vi "ToPythonVersionString.vi"(11 "Python版本":T1) -> (3 "python版本字符串":string)   [LabVIEW 2019]
doc: "将Python版本枚举转换为版本字符串的帮助VI，该字符串将用作“打开Python会话”节点的输入。"
uses:
  PythonVersionsEnum.ctl
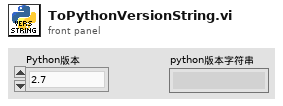
[diagram p1: front panel]
types:
  T1 = typedef "PythonVersionsEnum.ctl" = enum16{"2.7", "3.6"}
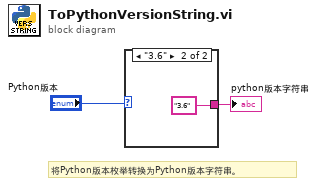
[diagram p0: block diagram]
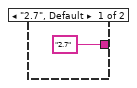
[diagram p2: hidden frame]
diagram:
  # "将Python版本枚举转换为Python版本字符串。"
  n1 = case shown="\"3.6\"" "Python版本" {
    tunnel: ["2.7" ("python version") "3.6" ("python version")] -> w1
    frame "2.7", Default {
    }
    frame "3.6" {
    }
  }
  "python版本字符串" <- w1
